vi "RMSetTracker.vi"(8 "error in (no error)":errorcluster, 10 "QTrk Instance":T1, 11 "ResultManager":T2={"InstancePtr"=0, "ResultManagerConfig"={"Number of beads"=0, "Number of frame info columns"=0, "Result scaling"={"X"=0.0, "Y"=0.0, "Z"=0.0}, "Result offset"={"X"=0.0, "Y"=0.0, "Z"=0.0}, "Write Interval"=100, "Max frames in memory"=100, "Binary output (1/0)"=0}}) -> (0 "error out":errorcluster, 3 "ResultManager (out)":T2={"InstancePtr"=0, "ResultManagerConfig"={"Number of beads"=0, "Number of frame info columns"=0, "Result scaling"={"X"=0.0, "Y"=0.0, "Z"=0.0}, "Result offset"={"X"=0.0, "Y"=0.0, "Z"=0.0}, "Write Interval"=100, "Max frames in memory"=100, "Binary output (1/0)"=0}})   [LabVIEW 2011]
uses:
  ResultManagerInstance.ctl
  ResultManagerConfig.ctl
  XYZf.ctl
  QTrkInstance.ctl
  QTrkDLL.vi
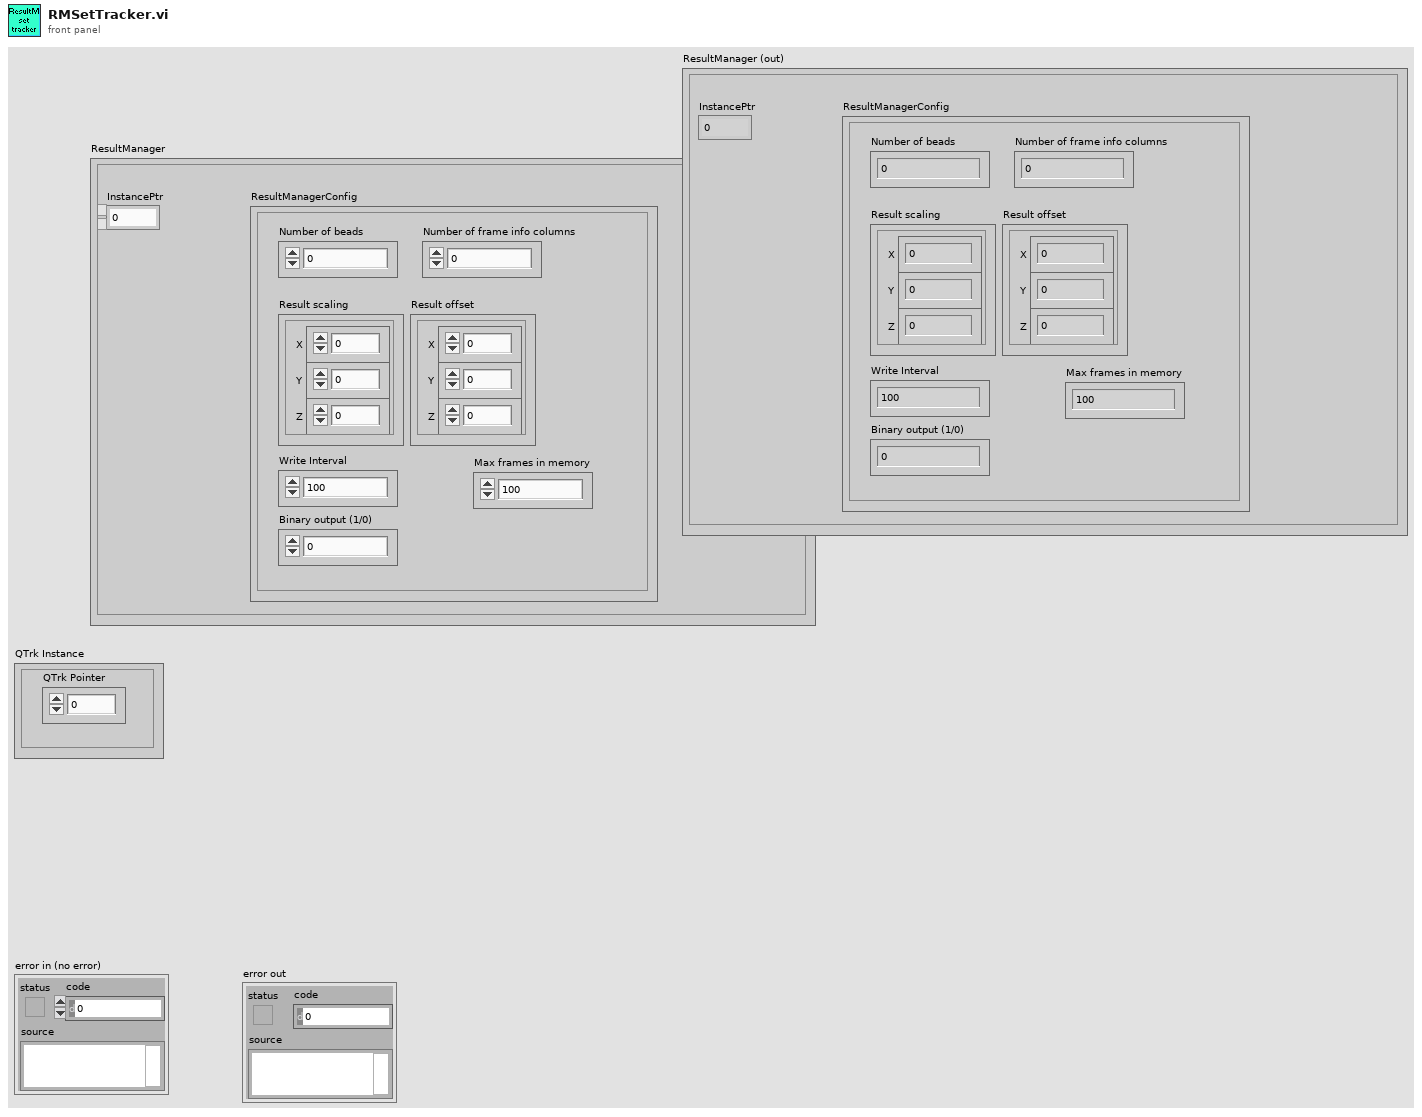
[diagram p1: front panel]
types:
  T1 = typedef "QTrkInstance.ctl" = cluster{"QTrk Pointer":u64}
  T2 = typedef "ResultManagerInstance.ctl" = cluster{"InstancePtr":u64, "ResultManagerConfig":T3}
  T3 = typedef "ResultManagerConfig.ctl" = cluster{"Number of beads":i32, "Number of frame info columns":i32, "Result scaling":T4, "Result offset":T4, "Write Interval":i32, "Max frames in memory":i32, "Binary output (1/0)":i8}
  T4 = typedef "XYZf.ctl" = cluster{"X":sgl, "Y":sgl, "Z":sgl}
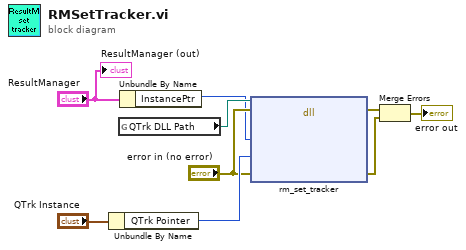
[diagram p0: block diagram]
diagram:
  n1 = Unbundle By Name("QTrk Instance") -> ("QTrk Pointer"=w7:u64)
  n2 = global read "QTrkDLL.vi" "QTrk DLL Path"() -> (w9:path)
  n3 = Unbundle By Name("ResultManager") -> ("InstancePtr"=w1:u64)
  n4 = dll-call lib="D:/jcnossen1/cudaqi-tracker/bin/jtrk-labview.dll" fn="rm_set_tracker"(path in=w9, error in="error in (no error)", "resultmanager"=w1, "qtrk"=w7, "err"="error in (no error)") -> (error out=w5:errorcluster, "err"=w4:errorcluster)  [unwired: 4 in, 1 out]
  n5 = Merge Errors(w5, w4) -> (→"error out":errorcluster)
  "ResultManager (out)" <- "ResultManager"
